vi "RSZVB Configure Sweep Time.vi"(6 "Sweep Time (21.91E-3 s)":dbl=0.021909 format="%^.3e", 7 "Meas Delay (0.0 s)":dbl format="%^.3e", 8 "error in (no error)":errorcluster {"code" format="%.0x"}, 9 "Auto Sweep Time (T: On)":bool=TRUE, 10 "Channel (1)":i32=1, 11 "VISA session":refnum<visa-resource-name>) -> (0 "error out":errorcluster {"code" format="%.0x"}, 3 "dup VISA session":refnum<visa-resource-name>)   [LabVIEW 2011]
doc: "This VI sets the measurement time for a sweep or delay the start of each sweep.\n\nNote(s):\n\nThe sweep duration is ignored for the sweep types Time and CW Mode.\n\nRemote-control command(s):\n[SENSe<Ch>:]SWEep:TIME:AUTO <Boolean>\n[SENSe<Ch>:]SWEep:TIME <numeric_value>\n[SENSe<Ch>:]SWEep:DWELl <numeric_value>"
panel:
  # "On\nOff"
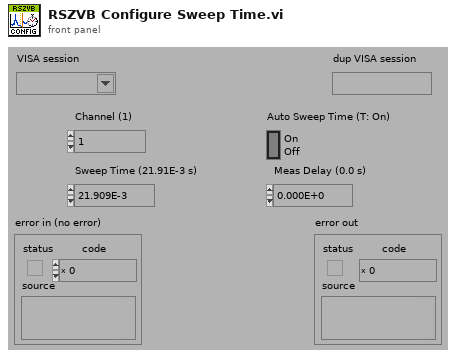
[diagram p1: front panel]
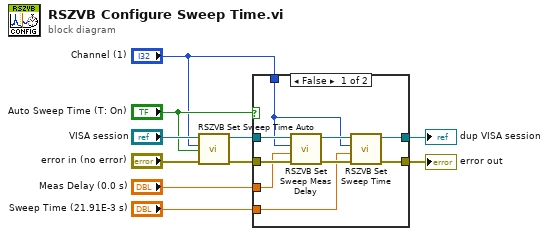
[diagram p0: block diagram]
diagram:
  n1 = call "RSZVB Set Sweep Time Auto.vi"("error in (no error)"="error in (no error)", "Auto Sweep Time (T: On)"="Auto Sweep Time (T: On)", "Channel (1)"="Channel (1)", "VISA session"="VISA session") -> ("error out"=w6:errorcluster, "dup VISA session"=w7:refnum<visa-resource-name>)  [unwired: 6 in]
  n2 = case shown="False" "Auto Sweep Time (T: On)" {
    tunnel: w7 -> [w19 w20]
    tunnel: w6 -> [w18 w21]
    tunnel: [w11 w21] -> w1
    tunnel: [w12 w20] -> w2
    tunnel: "Channel (1)" -> [w13 _]
    tunnel: "Meas Delay (0.0 s)" -> [w17 _]
    tunnel: "Sweep Time (21.91E-3 s)" -> [w14 _]
    frame False {
      n3 = call "RSZVB Set Sweep Meas Delay.vi"("error in (no error)"=w18, "Meas Delay (0.0 s)"=w17, "Channel (1)"=w13, "VISA session"=w19) -> ("error out"=w15:errorcluster, "dup VISA session"=w16:refnum<visa-resource-name>)  [unwired: 6 in]
      n4 = call "RSZVB Set Sweep Time.vi"("error in (no error)"=w15, "Sweep Time (21.909e-3 s)"=w14, "Channel (1)"=w13, "VISA session"=w16) -> ("error out"=w11:errorcluster, "dup VISA session"=w12:refnum<visa-resource-name>)  [unwired: 6 in]
    }
    frame True {
    }
  }
  "error out" <- w1
  "dup VISA session" <- w2
